vi "ReadBuffers.vi"(0 "VISA Refnum in":refnum<visa-resource-name>, 2 "Address":u8, 3 "error in (no error)":errorcluster) -> (1 "Buffer1":u8, 5 "Buffer2":u8, 6 "VISA Refnum out":refnum<visa-resource-name>, 7 "Valid":bool, 10 "error out":errorcluster)   [LabVIEW 2015, in "Ion Motion Roboclaw.lvlib"]
uses:
  <instrlib>/Ion Motion Roboclaw/Ion Motion Roboclaw.lvlib
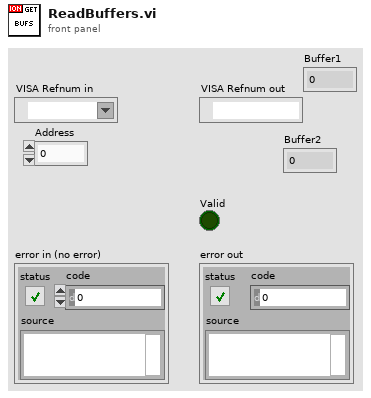
[diagram p1: front panel]
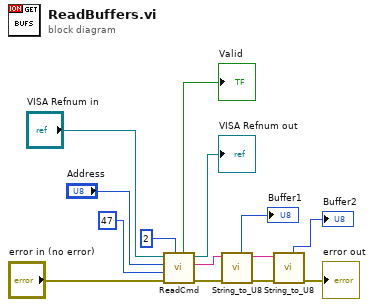
[diagram p0: block diagram]
diagram:
  n1 = call <instrlib>:"ReadCmd.vi"("Read Count"=u32 2, "error in (no error)"="error in (no error)", "Cmd"=u8 47, "Address"="Address", "VISA Refnum in"="VISA Refnum in") -> ("error out"=w6:errorcluster, "Output"=w5:string, "VISA Refnum out"=→"VISA Refnum out":refnum<visa-resource-name>, "Valid"=→"Valid":bool)  [unwired: 3 in]
  n2 = call <instrlib>:"String_to_U8.vi"("error in (no error)"=w6, "String"=w5) -> ("error out"=w13:errorcluster, "rest of the binary string"=w14:string, "Argument"=→"Buffer1":u8)  [unwired: 5 in]
  n3 = call <instrlib>:"String_to_U8.vi"("error in (no error)"=w13, "String"=w14) -> ("error out"=→"error out":errorcluster, "Argument"=→"Buffer2":u8)  [unwired: 5 in, 1 out]
